vi "BasicAlgebra.vi"() -> ()   [LabVIEW 2019]
panel:
  in  "Ring":u16(ring) items=["Add", "Subtract", "Multiply", "Divide"]
  in  "stop":bool
  out "result":dbl
  in  "num2":dbl
  in  "num1":dbl
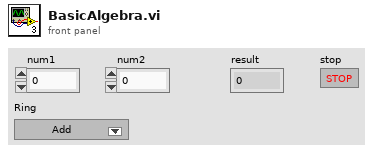
[diagram p1: front panel]
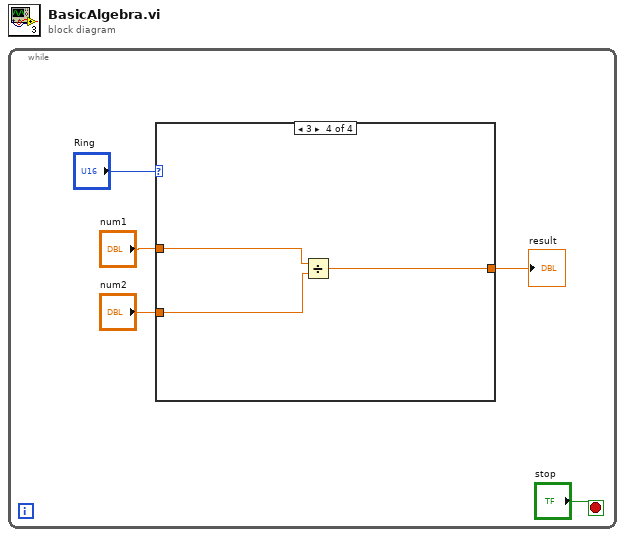
[diagram p0: block diagram]
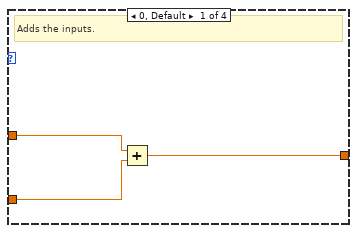
[diagram p2: hidden frame]
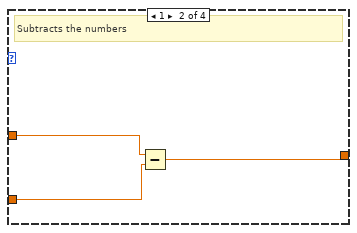
[diagram p3: hidden frame]
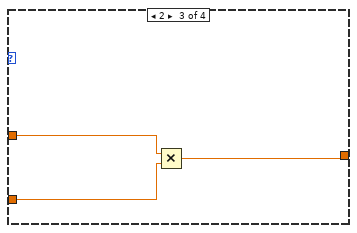
[diagram p4: hidden frame]
diagram:
  n1 = while {
    stop <- "stop" stop-if-true
    n2 = case shown="3" "Ring" {
      tunnel: "num1" -> [w8 w11 w14 w17]
      tunnel: "num2" -> [w7 w10 w13 w16]
      tunnel: [w6 w9 w12 w15] -> w1
      frame 0, Default {
        # "Adds the inputs."
        n3 = Add(x=w8, y=w7) -> (x+y=w6:dbl)
      }
      frame 1 {
        # "Subtracts the numbers"
        n4 = Subtract(x=w11, y=w10) -> (x-y=w9:dbl)
      }
      frame 2 {
        n5 = Multiply(x=w14, y=w13) -> (x*y=w12:dbl)
      }
      frame 3 {
        n6 = Divide(x=w17, y=w16) -> (x/y=w15:dbl)
      }
    }
    "result" <- w1
  }
